vi "select spot when imaging.vi"(10 "current location":T3, 11 "spot location constraints":T4=[{"spot number"=0, "active"=FALSE, "x max"=0, "x min"=0, "y max"=0, "y min"=0}, {"spot number"=0, "active"=FALSE, "x max"=0, "x min"=0, "y max"=0, "y min"=0}, {"spot number"=0, "active"=FALSE, "x max"=0, "x min"=0, "y max"=0, "y min"=0}, {"spot number"=0, "active"=FALSE, "x max"=0, "x min"=0, "y max"=0, "y min"=0}]) -> (0 "update tracking?":T1, 1 "acquire":bool, 3 "selected spot":T2)   [LabVIEW 2010]
uses:
  spot location constraints.ctl
  spot location constraint.ctl
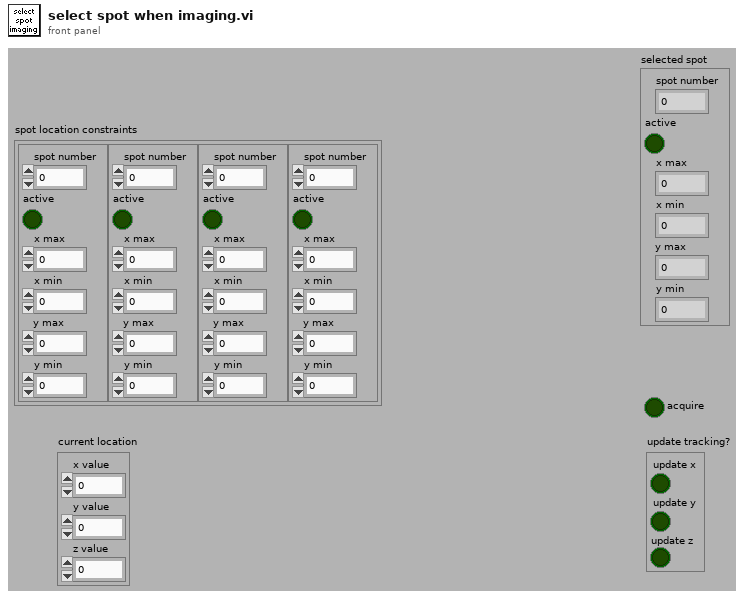
[diagram p1: front panel]
types:
  T1 = cluster{"update x":bool, "update y":bool, "update z":bool}
  T2 = typedef "spot location constraint.ctl" = cluster{"spot number":i8, "active":bool, "x max":i16, "x min":i16, "y max":i16, "y min":i16}
  T3 = cluster{"x value":i16, "y value":i16, "z value":i16}
  T4 = typedef "spot location constraints.ctl" = T2[]
  T5 = cluster{"crossing":bool, "crossing":bool, "crossing":bool}
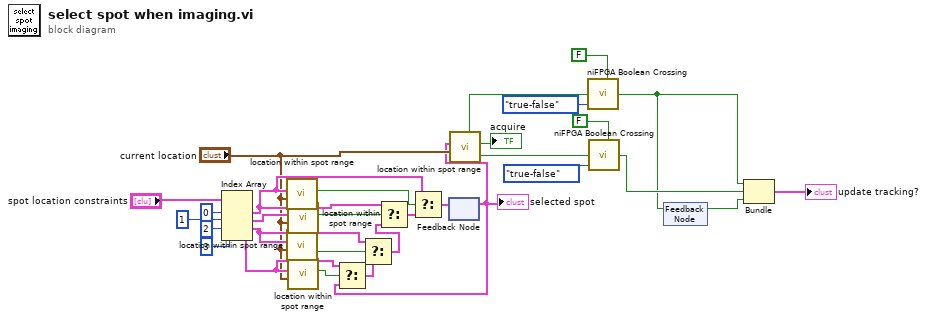
[diagram p0: block diagram]
diagram:
  n1 = Index Array(array="spot location constraints", index #1=0 ("index"), index #2=1 ("index"), index #3=2 ("index"), index #4=3 ("index")) -> (element #1=w15:T2, element #2=w25:T2, element #3=w20:T2, element #4=w23:T2)
  n2 = call "location within spot range"("current location"="current location", "spot location constraint"=w15) -> ("spot selected"=w16:bool)  [unwired: 7 in, 2 out]
  n3 = call "location within spot range"("current location"="current location", "spot location constraint"=w20) -> ("spot selected"=w21:bool)  [unwired: 7 in, 2 out]
  n4 = call "location within spot range"("current location"="current location", "spot location constraint"=w25) -> ("spot selected"=w19:bool)  [unwired: 7 in, 2 out]
  n5 = call "location within spot range"("current location"="current location", "spot location constraint"=w23) -> ("spot selected"=w24:bool)  [unwired: 7 in, 2 out]
  n6 = feedback #1() -> (w8:T2)  [unwired: 1 in]
  "selected spot" <- w8
  n7 = Select(t=w23, s=w24, f=w8) -> (s? t:f=w22:T2)
  n8 = Select(t=w20, s=w21, f=w22) -> (s? t:f=w18:T2)
  n9 = Select(t=w15, s=w19, f=w18) -> (s? t:f=w17:T2)
  n10 = Select(t=w15, s=w16, f=w17) -> (s? t:f=w14:T2)
  n11 = feedback-in #1(w14) -> ()
  n12 = call "location within spot range"("current location"="current location", "spot location constraint"=w8) -> ("spot selected"=→"acquire":bool, "y-valid"=w7:bool, "x-valid"=w11:bool)  [unwired: 7 in]
  n13 = call <vilib>:"niFPGA Boolean Crossing.vi"("input"=w11, "direction"=enum8{"either", "false-true", "true-false"}."true-false", "initialize"=FALSE) -> ("crossing"=w2:bool)  [unwired: 6 in]
  n14 = call <vilib>:"niFPGA Boolean Crossing.vi"("input"=w7, "direction"=enum8{"either", "false-true", "true-false"}."true-false", "initialize"=FALSE) -> ("crossing"=w3:bool)  [unwired: 6 in]
  n15 = feedback-in #2(w2) -> ()
  n16 = feedback #2() -> (w4:bool)  [unwired: 1 in]
  n17 = Bundle("crossing"=w2, "crossing"=w3, "crossing"=w4) -> (→"update tracking?":T5)  [unwired: 1 in]
